vi "RT_test2.vi"() -> ()   [LabVIEW 2018]
panel:
  in  "stop":bool
  out "loop2":i32
  out "loop1":i32
  out "dt":u32
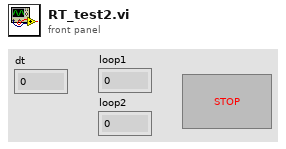
[diagram p1: front panel]
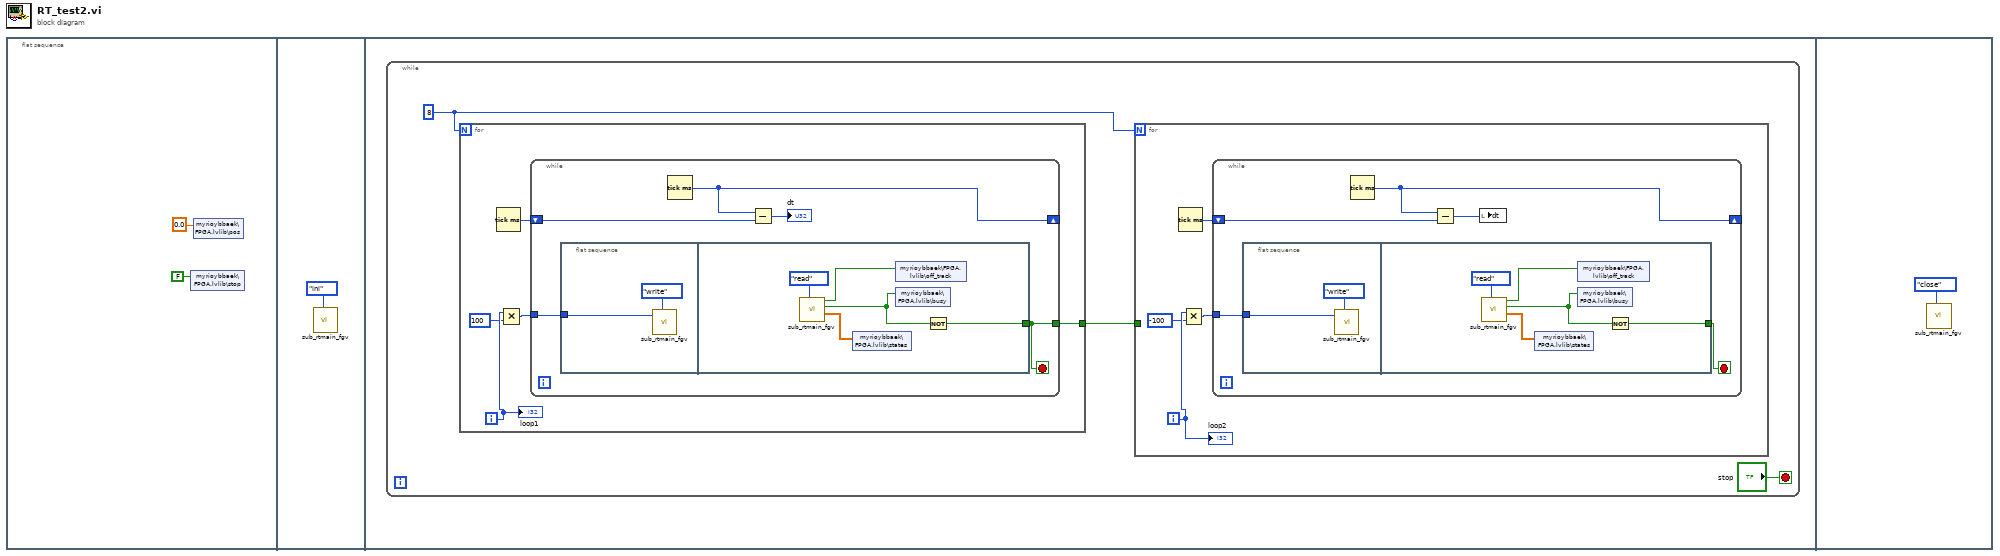
[diagram p0: block diagram]
diagram:
  n1 = flat-sequence {
    frame #0 {
      n2 = shared-variable "myrioybbaek\\FPGA.lvlib\\stop"(FALSE ("stop")) -> ()  [unwired: 1 in, 1 out]
      n3 = shared-variable "myrioybbaek\\FPGA.lvlib\\pos"(0.0 ("pos")) -> ()  [unwired: 1 in, 1 out]
    }
    frame #1 {
      n4 = call "sub_rtmain_fgv.vi"("cmd"=enum16{"ini", "read", "write", "close"}."ini") -> ()  [unwired: 7 in, 4 out]
    }
    frame #2 {
      n5 = while {
        stop <- "stop" stop-if-true
        w5 = 8
        n6 = for {
          N: w5 -> [_]
          tunnel: [w23] -> w6
          i -> [w26]
          n7 = Tick Count (ms)() -> (millisecond timer value=w27:u32)
          n8 = Multiply(x=w26, y=100) -> (x*y=w24:i32)
          n9 = while {
            shift-right: [w32] -> _
            shift-left: w27 -> [w31]
            tunnel: w24 -> [w29]
            tunnel: [w28] -> w23
            stop <- w28 stop-if-true
            n10 = flat-sequence {
              tunnel: w29 -> [w33]
              tunnel: [w35] -> w28
              frame #0 {
                n11 = call "sub_rtmain_fgv.vi"("cmd"=enum16{"ini", "read", "write", "close"}."write", "setpoint"=w33) -> ()  [unwired: 6 in, 4 out]
              }
              frame #1 {
                n12 = call "sub_rtmain_fgv.vi"("cmd"=enum16{"ini", "read", "write", "close"}."read") -> ("states"=w39:dbl[], "busy"=w36:bool, "off_track"=w37:bool)  [unwired: 7 in, 1 out]
                n13 = shared-variable "myrioybbaek\\FPGA.lvlib\\states"(w39) -> ()  [unwired: 1 in, 1 out]
                n14 = shared-variable "myrioybbaek\\FPGA.lvlib\\off_track"(w37) -> ()  [unwired: 1 in, 1 out]
                n15 = shared-variable "myrioybbaek\\FPGA.lvlib\\busy"(w36) -> ()  [unwired: 1 in, 1 out]
                n16 = Not(x=w36) -> (.not. x?=w35:bool)
              }
            }
            n17 = Tick Count (ms)() -> (millisecond timer value=w32:u32)
            n18 = Subtract(x=w32, y=w31) -> (x-y=→"dt":u32)
          }
          "loop1" <- w26
        }
        n19 = for {
          N: w5 -> [_]
          tunnel: w6 -> [_]
          i -> [w9]
          n20 = Tick Count (ms)() -> (millisecond timer value=w10:u32)
          n21 = Multiply(x=w9, y=-100) -> (x*y=w7:i32)
          n22 = while {
            shift-right: [w15] -> _
            shift-left: w10 -> [w14]
            tunnel: w7 -> [w12]
            stop <- w13 stop-if-true
            n23 = flat-sequence {
              tunnel: w12 -> [w16]
              tunnel: [w18] -> w13
              frame #0 {
                n24 = call "sub_rtmain_fgv.vi"("cmd"=enum16{"ini", "read", "write", "close"}."write", "setpoint"=w16) -> ()  [unwired: 6 in, 4 out]
              }
              frame #1 {
                n25 = call "sub_rtmain_fgv.vi"("cmd"=enum16{"ini", "read", "write", "close"}."read") -> ("states"=w22:dbl[], "busy"=w19:bool, "off_track"=w20:bool)  [unwired: 7 in, 1 out]
                n26 = shared-variable "myrioybbaek\\FPGA.lvlib\\states"(w22) -> ()  [unwired: 1 in, 1 out]
                n27 = shared-variable "myrioybbaek\\FPGA.lvlib\\off_track"(w20) -> ()  [unwired: 1 in, 1 out]
                n28 = shared-variable "myrioybbaek\\FPGA.lvlib\\busy"(w19) -> ()  [unwired: 1 in, 1 out]
                n29 = Not(x=w19) -> (.not. x?=w18:bool)
              }
            }
            n30 = Tick Count (ms)() -> (millisecond timer value=w15:u32)
            n31 = Subtract(x=w15, y=w14) -> (x-y=w11:u32)
            n32 = local write "dt"(w11) -> ()
          }
          "loop2" <- w9
        }
      }
    }
    frame #3 {
      n33 = call "sub_rtmain_fgv.vi"("cmd"=enum16{"ini", "read", "write", "close"}."close") -> ()  [unwired: 7 in, 4 out]
    }
  }
